vi "DraggingDresser.vi"() -> ()   [LabVIEW 2015]
panel:
  out "Force":dbl[](array[numeric])
  out "Angle for Minimum Force":i32 format="%.1f"
  in  "Coefficient of Kinetic Friction":dbl format="%.1f"
  out "Waveform Graph":dbl[](graph)
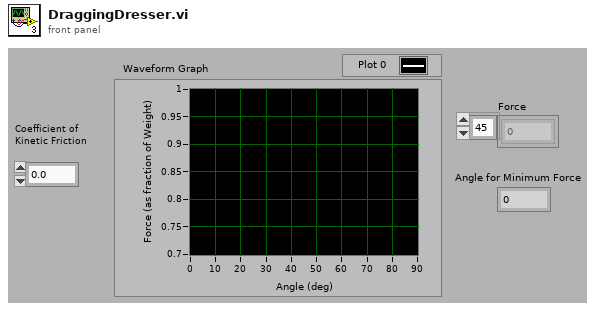
[diagram p1: front panel]
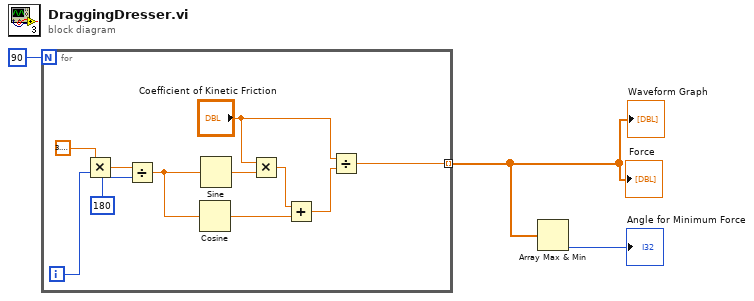
[diagram p0: block diagram]
diagram:
  n1 = for {
    N: 90 -> [_]
    tunnel: [w4] -> w2 mode=indexing
    i -> [w5]
    n2 = Multiply(x=3.141592653589793, y=w5) -> (x*y=w13:dbl)
    n3 = Divide(x=w13, y=180) -> (x/y=w11:dbl)
    n4 = Cosine(x=w11) -> (cos(x)=w8:dbl)
    n5 = Sine(x=w11) -> (sin(x)=w10:dbl)
    n6 = Multiply(x="Coefficient of Kinetic Friction", y=w10) -> (x*y=w9:dbl)
    n7 = Add(x=w9, y=w8) -> (x+y=w6:dbl)
    n8 = Divide(x="Coefficient of Kinetic Friction", y=w6) -> (x/y=w4:dbl)
  }
  "Waveform Graph" <- w2
  "Force" <- w2
  n9 = Array Max & Min(array=w2) -> (min index (indices)=→"Angle for Minimum Force":i32)  [unwired: 3 out]
